vi "SSI_Initialize.vi"(0 "VISA resource name":refnum<visa-resource-name>, 5 "Remote Mode":u16(ring) items=["USB", "RS232", "GPIB", "Ethernet"], 7 "baud rate (921600)":u32=921600, 9 "Ethernet":T1={"Port"=10001.0, "Timeout"=1000, "IP Address"=""}, 11 "error in (no error)":errorcluster) -> (4 "VISA resource name out":refnum<visa-resource-name>, 6 "connection ID(Ethernet)":refnum<k5>, 15 "error out":errorcluster)   [LabVIEW 2019]
uses:
  <vilib>/Instr/_visa.llb/VISA Set IO Buffer Mask.ctl
  <vilib>/Instr/_visa.llb/VISA Configure Serial Port (Instr).vi
panel:
  # "USB/RS232"
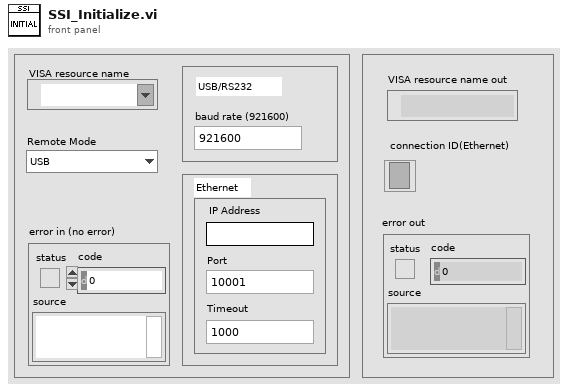
[diagram p1: front panel]
types:
  T1 = cluster{"Port":dbl, "Timeout":u16, "IP Address":string}
  T2 = typedef "VISA Set IO Buffer Mask.ctl" = u16
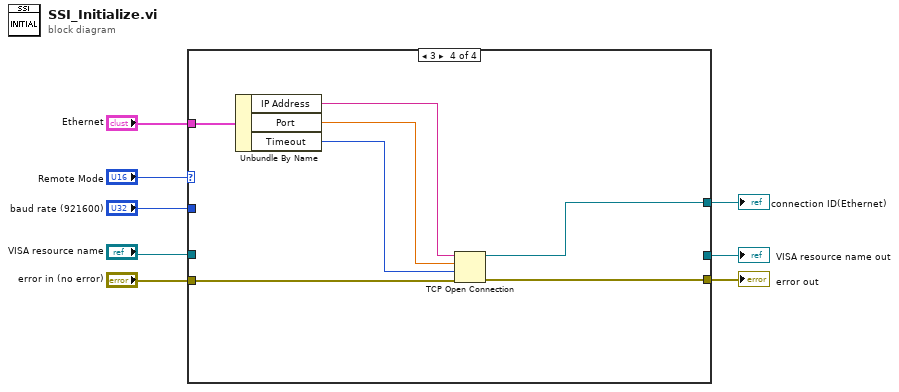
[diagram p0: block diagram]
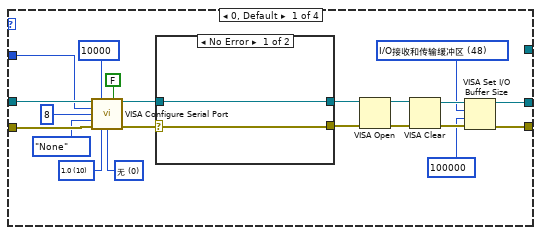
[diagram p2: hidden frame]
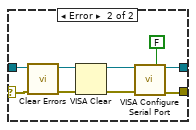
[diagram p3: hidden frame]
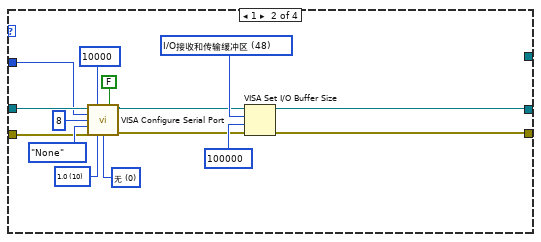
[diagram p4: hidden frame]
diagram:
  n1 = case shown="3" "Remote Mode" {
    tunnel: "VISA resource name" -> [w27 w48 w56 _]
    tunnel: "error in (no error)" -> [w26 w47 w55 w63]
    tunnel: "baud rate (921600)" -> [w13 w46 _ _]
    tunnel: [w16 w44 w56 _] -> w4
    tunnel: [w15 w43 w55 w62] -> w3
    tunnel: [_ _ _ w61] -> w2
    tunnel: "Ethernet" -> [_ _ _ w60]
    frame 0, Default {
      w14 = T2 48 items=["I/O接收缓冲区"=16, "I/O传输缓冲区"=32, "I/O接收和传输缓冲区"=48] ("Mask")
      w21 = u16 0 items=["无", "XON/XOFF", "RTS/CTS", "XON/XOFF & RTS/CTS", "DTR/DSR", "XON/XOFF & DTR/DSR"] ("flow control (0:none)")
      w22 = u16 10 items=["1.0"=10, "1.5"=15, "2.0"=20] ("stop bits (10: 1 bit)")
      n2 = call-poly "VISA Configure Serial Port"("VISA resource name"=w27, "timeout (10sec)"=u32 10000, "Enable Termination\nChar (T)"=FALSE ("Enable Termination\nChar (T)"), "baud rate (9600)"=w13, "data bits (8)"=u16 8, "parity (0:none)"=enum16{"None", "Odd", "Even", "Mark", "Space"}."None", "error in (no error)"=w26, "stop bits (10: 1 bit)"=w22, "flow control (0:none)"=w21) -> ("VISA resource name out"=w11:refnum<visa-resource-name>, "error out"=w12:errorcluster)  [unwired: 5 in]
      n3 = case shown="No Error" w12 {
        selector: w12 -> [w31 w38]
        tunnel: w11 -> [w30 w33]
        tunnel: [w31 w36] -> w10
        tunnel: [w30 w35] -> w9
        frame No Error {
        }
        frame Error {
          n4 = call <vilib>:"Clear Errors.vi"("error in (no error)"=w38) -> ("error out"=w39:errorcluster)  [unwired: 5 in, 1 out]
          n5 = VISA Clear(VISA resource name=w33, error in (no error)=w39) -> (VISA resource name out=w34:refnum<visa-resource-name>, error out=w37:errorcluster)
          n6 = call-poly "VISA Configure Serial Port"("VISA resource name"=w34, "Enable Termination\nChar (T)"=FALSE ("Enable Termination\nChar (T)"), "error in (no error)"=w37) -> ("VISA resource name out"=w35:refnum<visa-resource-name>, "error out"=w36:errorcluster)  [unwired: 11 in]
        }
      }
      n7 = VISA Open(error in (no error)=w10, VISA resource name=w9) -> (VISA resource name=w29:refnum<visa-resource-name>, error out=w28:errorcluster)  [unwired: 3 in]
      n8 = VISA Clear(VISA resource name=w29, error in (no error)=w28) -> (VISA resource name out=w19:refnum<visa-resource-name>, error out=w18:errorcluster)
      n9 = VISA Set I/O Buffer Size(VISA resource name=w19, mask (16)=w14, size (4096)=u32 100000 ("大小(4096)"), error in (no error)=w18) -> (VISA resource name out=w16:refnum<visa-resource-name>, error out=w15:errorcluster)
    }
    frame 1 {
      w42 = T2 48 items=["I/O接收缓冲区"=16, "I/O传输缓冲区"=32, "I/O接收和传输缓冲区"=48] ("Mask")
      w50 = u16 0 items=["无", "XON/XOFF", "RTS/CTS", "XON/XOFF & RTS/CTS", "DTR/DSR", "XON/XOFF & DTR/DSR"] ("flow control (0:none)")
      w51 = u16 10 items=["1.0"=10, "1.5"=15, "2.0"=20] ("stop bits (10: 1 bit)")
      n10 = call-poly "VISA Configure Serial Port"("VISA resource name"=w48, "timeout (10sec)"=u32 10000, "Enable Termination\nChar (T)"=FALSE ("Enable Termination\nChar (T)"), "baud rate (9600)"=w46, "data bits (8)"=u16 8, "parity (0:none)"=enum16{"None", "Odd", "Even", "Mark", "Space"}."None", "error in (no error)"=w47, "stop bits (10: 1 bit)"=w51, "flow control (0:none)"=w50) -> ("VISA resource name out"=w41:refnum<visa-resource-name>, "error out"=w40:errorcluster)  [unwired: 5 in]
      n11 = VISA Set I/O Buffer Size(VISA resource name=w41, mask (16)=w42, size (4096)=u32 100000 ("大小(4096)"), error in (no error)=w40) -> (VISA resource name out=w44:refnum<visa-resource-name>, error out=w43:errorcluster)
    }
    frame 2 {
    }
    frame 3 {
      n12 = Unbundle By Name(w60) -> ("IP Address"=w57:string, "Port"=w59:dbl, "Timeout"=w58:u16)
      n13 = TCP Open Connection(address=w57, remote port or service name=w59, timeout ms (60000)=w58, error in (no error)=w63) -> (connection ID=w61:refnum<k5>, error out=w62:errorcluster)  [unwired: 1 in]
    }
  }
  "error out" <- w3
  "VISA resource name out" <- w4
  "connection ID(Ethernet)" <- w2
